vi "CreatePublicEvents.vi"(8 "error in (no error)":errorcluster, 11 "Inst.Transport":refnum<class "Inst.Transport.lvclass">) -> (0 "error out":errorcluster, 3 "Inst.Transport out":refnum<class "Inst.Transport.lvclass">)   [LabVIEW 2019, in "Inst.Transport.lvclass"]
doc: "---------------------------------------------------------------\nJKI State Machine Objects™\nhttp://jki.net/state-machine-objects/\nCopyright (C) 2005-2015, JKI <info@jki.net>\nALL RIGHTS RESERVEDJKI State Machine Objects (SMO) 1.0.0.4\nJKI - JKI\nCopyright (c) 2015, JKI"
uses:
  Inst.Transport.lvclass
  <userlib>/LevyLab/Instrument Framework/Instrument Types/SCPI/Instrument.SCPI.lvclass
  Typedefs/UI State--enum.ctl
panel:
  # "For instructions on how to use the JKI State Machine Objects, examples and video tutorials, visit:\nhttp://jki.net/state-machine-objects/\n\nJKI State Machine Objects™\nhttp://jki.net/state-machine-objects/\nCopyright (C) 2005-2015, JKI <info@jki.net>\nALL RIGHTS RESERVED"
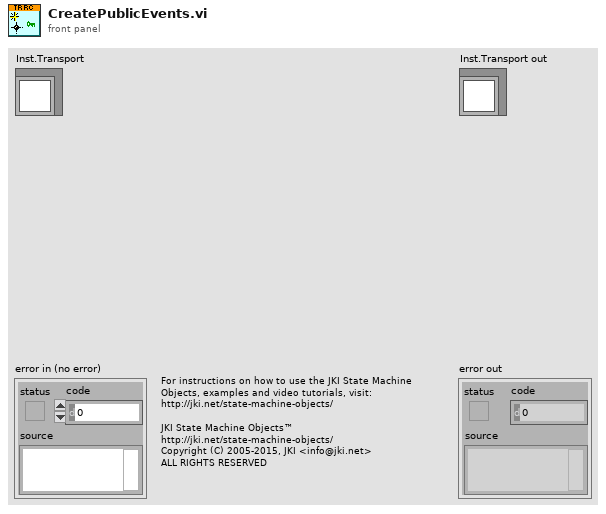
[diagram p1: front panel]
types:
  T1 = typedef "Inst.Transport.lvclass/UI State--enum.ctl" = enum16{"unknown", "Opened", "Closed"}
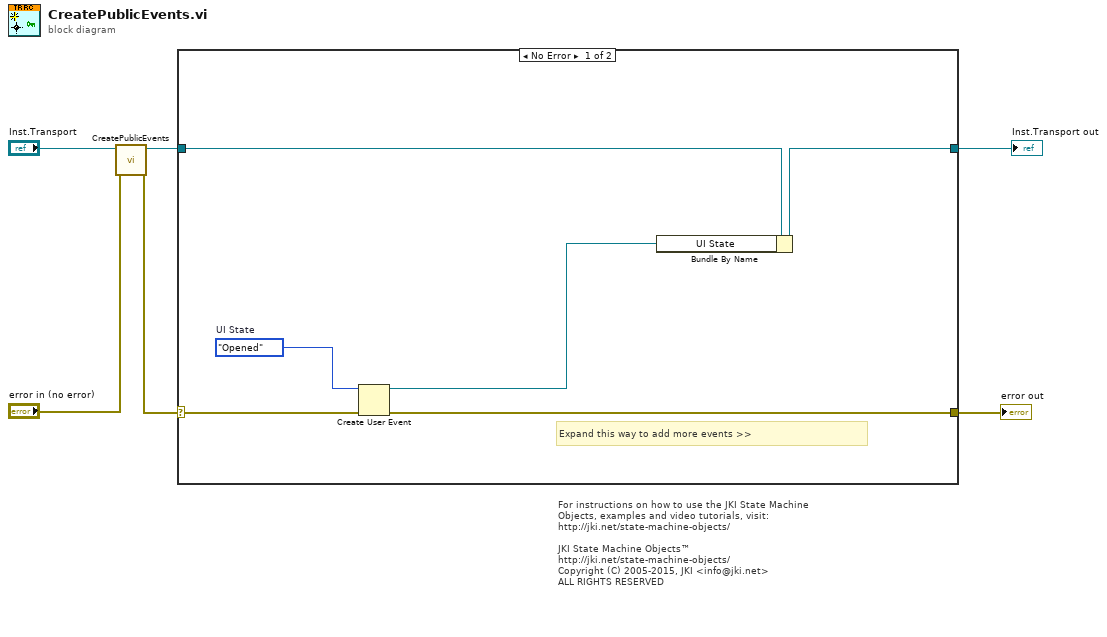
[diagram p0: block diagram]
diagram:
  # "For instructions on how to use the JKI State Machine Objects, examples and video tutorials, visit:\nhttp://jki.net/state-machine-objects/\n\nJKI State Machine Objects™\nhttp://jki.net/state-machine-objects/\nCopyright (C) 2005-2015, JKI <info@jki.net>\nALL RIGHTS RESERVED"
  n1 = call-parent "CreatePublicEvents.vi"("error in (no error)"="error in (no error)", "Instrument"="Inst.Transport") -> ("error out"=w1:errorcluster, "Instrument out"=w5:refnum<class "Inst.Transport.lvclass">)  [unwired: 8 in]
  n2 = case shown="No Error" w1 {
    selector: w1 -> [w12 w14]
    tunnel: [w11 w14] -> w3
    tunnel: [w8 w13] -> w4
    tunnel: w5 -> [w7 w13]
    frame No Error {
      w10 = UI_State--enum."Opened"  # UI State
      # "Expand this way to add more events >>"
      n3 = Create User Event(user event datatype=w10, error in=w12) -> (user event=w9:refnum<user-event>, error out=w11:errorcluster)
      n4 = Bundle By Name(cluster=w7, "UI State"=w9) -> (w8:refnum<class "Inst.Transport.lvclass">)
    }
    frame Error {
    }
  }
  "error out" <- w3
  "Inst.Transport out" <- w4
